vi "globalTearDown.vi"(8 "error in (no error)":errorcluster, 11 "Single Core Simple Loopback in":refnum<class "Single Board 1Ch Loopback.lvclass">) -> (0 "error out":errorcluster, 3 "Single Core Simple Loopback out":refnum<class "Single Board 1Ch Loopback.lvclass">)   [LabVIEW 2020, in "Single Board 1Ch Loopback.lvclass"]
uses:
  Single Board 1Ch Loopback.lvclass
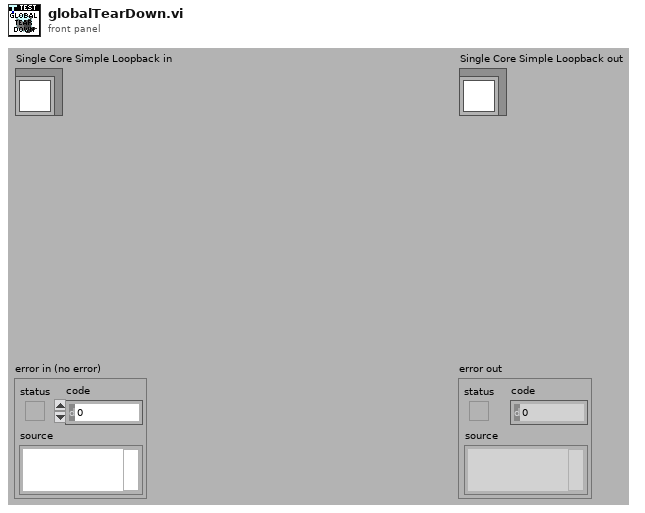
[diagram p1: front panel]
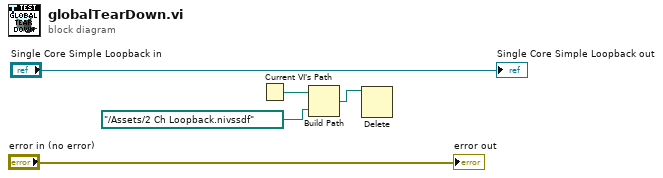
[diagram p0: block diagram]
diagram:
  n1 = Current VI's Path() -> (path=w3:path)
  n2 = Build Path(base path=w3, name or relative path=path "../Assets/2 Ch Loopback.nivssdf" ("Hardware File Path")) -> (appended path=w1:path)
  n3 = Delete(path (use dialog)=w1) -> ()  [unwired: 4 in, 3 out]
  "error out" <- "error in (no error)"
  "Single Core Simple Loopback out" <- "Single Core Simple Loopback in"
